vi "XY Graph Fold Plot.vi"(6 "# Folds (1)":u32=1, 8 "error in (no error)":errorcluster, 9 "Replace Plot (T)?":bool=TRUE, 11 "Selected Plot Info":T1={"Multiplot XY Graph"=refnum, "Mouse Coordinates"={"Horizontal"=0, "Vertical"=0}, "Plot Index"=-1}) -> (0 "Error Out":errorcluster, 1 "Fold Decay Message":string, 3 "Folded Decay":cluster{"t Array":dbl[], "IRF Array":dbl[]})   [LabVIEW 2021, in "XY Graph Add-Ons.lvlib"]
uses:
  XY Graph Selected Plot Info.ctl
  XY Graph Refnum.ctl
  <vilib>/Utility/miscctls.llb/LVPoint32TypeDef.ctl
  XY Graph Add-Ons.lvlib
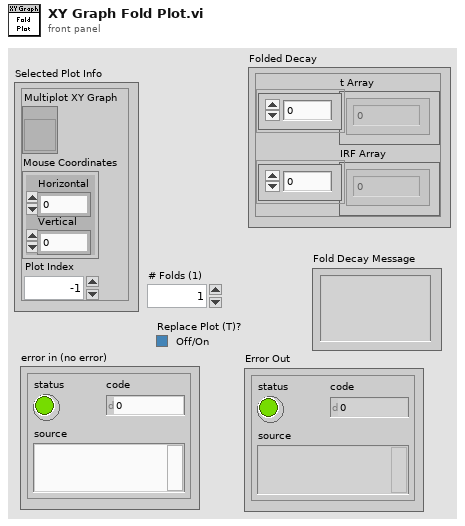
[diagram p1: front panel]
types:
  T1 = typedef "XY Graph Add-Ons.lvlib/XY Graph Selected Plot Info.ctl" = cluster{"Multiplot XY Graph":T2, "Mouse Coordinates":T3, "Plot Index":i32}
  T2 = typedef "XY Graph Add-Ons.lvlib/XY Graph Refnum.ctl" = refnum<vi>
  T3 = typedef "LVPoint32TypeDef.ctl" = cluster{"Horizontal":i32, "Vertical":i32}
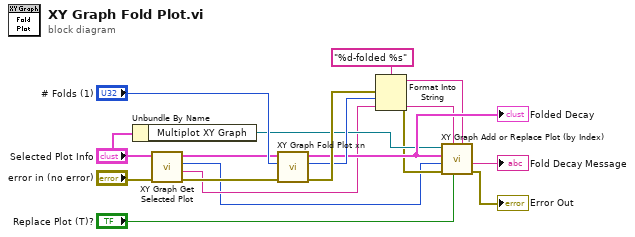
[diagram p0: block diagram]
diagram:
  n1 = Unbundle By Name("Selected Plot Info") -> ("Multiplot XY Graph"=w8:T2)
  n2 = call "XY Graph Get Selected Plot.vi"("error in (no error)"="error in (no error)", "Selected Plot Info"="Selected Plot Info") -> ("error out"=w11:errorcluster, "Plot Name"=w4:string, "Plot Index"=w1:i32, "Plot"=w12:cluster{"X Array":dbl[], "Y Array":dbl[]})  [unwired: 4 in, 2 out]
  n3 = call "XY Graph Fold Plot xn.vi"("Error In"=w11, "# Folds"="# Folds (1)", "Decay (in) in"=w12) -> ("Error Out"=w15:errorcluster, "# Folds (actual)"=w14:u32, "Decay (in) out"=w9:cluster{"X Axis":dbl[], "Y Axis":dbl[]})  [unwired: 5 in, 1 out]
  "Folded Decay" <- w9
  n4 = Format Into String(format string="%d-folded %s", error in=w15, w14, w4) -> (resulting string=w3:string, error out=w7:errorcluster)  [unwired: 1 in]
  n5 = call "XY Graph Add or Replace Plot (by Index).vi"("New Plot Name"=w3, "Replace Plot (T)?"="Replace Plot (T)?", "Original Plot Name"=w4, "error in (no error)"=w7, "Plot Index"=w1, "Plot in"=w9, "XYGraph in"=w8) -> ("error out"=→"Error Out":errorcluster, "Message"=→"Fold Decay Message":string)  [unwired: 3 in]
